vi "数据插入数据库.vi"(8 "error in (no error)":errorcluster, 9 "data输出":T1={"时间标识"=timestamp(0 s since 1904-01-01), "测量模式"="水样测试", "数据类型"="N", "监测值"=0.0, "单位"="mg/L", "数据标识"="N", "因子编码"=""}, 10 "table 输入":string, 11 "database":string="database1.mdb") -> (0 "error out":errorcluster)   [LabVIEW 2016, in "流量计.lvlib"]
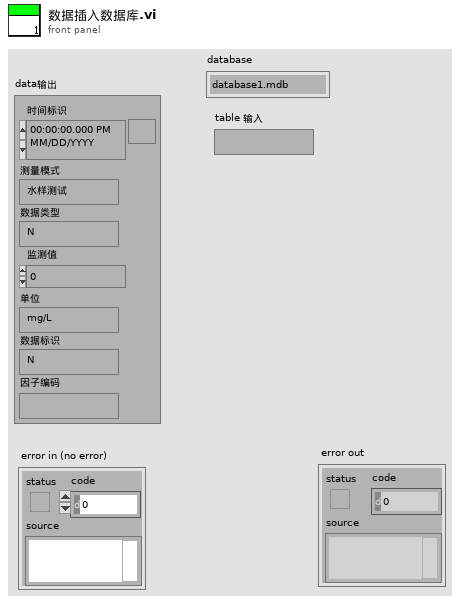
[diagram p1: front panel]
types:
  T1 = cluster{"时间标识":timestamp, "测量模式":string, "数据类型":string, "监测值":sgl, "单位":string, "数据标识":string, "因子编码":string}
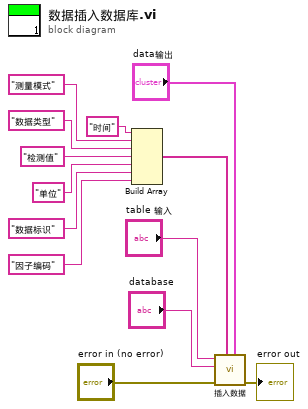
[diagram p0: block diagram]
diagram:
  n1 = Build Array("时间", "测量模式", "数据类型", "检测值", "单位", "数据标识", "因子编码") -> (w4:string[])
  n2 = call "插入数据.vi"("data"="data输出", "columns"=w4, "error in (no error)"="error in (no error)", "database"="database", "table"="table 输入") -> ("error out"=→"error out":errorcluster)  [unwired: 6 in]
